vi "CreateRotationY.vi"(8 "error in (no error)":errorcluster, 9 "radians":sgl, 11 "3D Scene in":refnum<class "3D Scene.lvclass">) -> (0 "error out":errorcluster, 2 "modelview rotated":T1, 3 "3D Scene out":refnum<class "3D Scene.lvclass">)   [LabVIEW 2015, in "3D Scene.lvclass"]
uses:
  3D Scene.lvclass
  <vilib>/Analysis/Matrix/Datatypes/RealMatrix.ctl
  <vilib>/Analysis/Matrix/NI_Matrix.lvlib
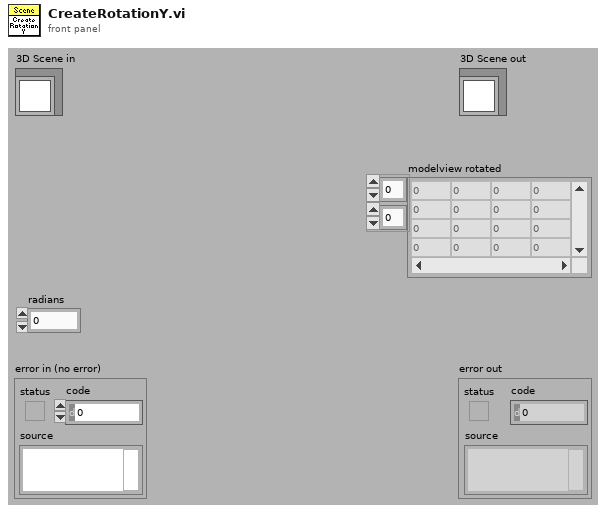
[diagram p1: front panel]
types:
  T1 = typedef "NI_Matrix.lvlib/RealMatrix.ctl" = dbl[][]
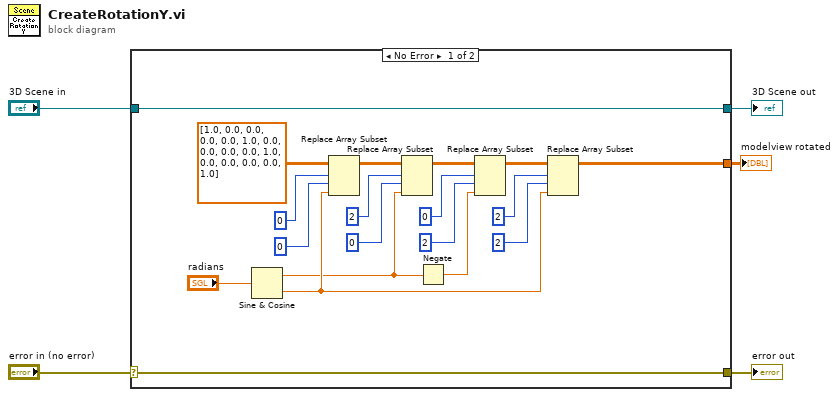
[diagram p0: block diagram]
diagram:
  n1 = case shown="No Error" "error in (no error)" {
    selector: "error in (no error)" -> [w23 w26]
    tunnel: [w23 w26] -> w4
    tunnel: [w24 w25] -> w2
    tunnel: "3D Scene in" -> [w24 w25]
    tunnel: [w9 _] -> w1
    frame No Error {
      n2 = Sine & Cosine(0:"radians") -> (1:w7:sgl, 2:w21:sgl)
      n3 = Replace Array Subset(array=T1 [[1.0, 0.0, 0.0, 0.0], [0.0, 1.0, 0.0, 0.0], [0.0, 0.0, 1.0, 0.0], [0.0, 0.0, 0.0, 1.0]] ("A"), new element=w21, index (row)=0, index (col)=0 ("disabled index (col)")) -> (w10:T1)
      n4 = Replace Array Subset(array=w10, new element=w7, index (row)=2 ("disabled index (row)"), index (col)=0 ("disabled index (col)")) -> (w11:T1)
      n5 = Negate(x=w7) -> (-x=w8:sgl)
      n6 = Replace Array Subset(array=w11, new element=w8, index (row)=0, index (col)=2 ("disabled index (col)")) -> (w12:T1)
      n7 = Replace Array Subset(array=w12, new element=w21, index (row)=2, index (col)=2 ("disabled index (col)")) -> (w9:T1)
    }
    frame Error {
    }
  }
  "error out" <- w4
  "3D Scene out" <- w2
  "modelview rotated" <- w1
